vi "Termostato1.vi"() -> ()   [LabVIEW 2023]
uses:
  <vilib>/measure/NI_MABase.lvlib
panel:
  out "Coste del \nsuministro":dbl
  out "Potencia de \nla calefacción":dbl
  out "Consumo":bool
  out "Diferencia de temperatura":waveform(dbl)(graph)
  in  "offset":dbl format="%0.2p"
  in  "frequency":dbl=10.0 format="%0.2p"
  in  "amplitude":dbl=1.0 format="%0.2p"
  out "Temperatura\n Deseada":dbl format="%#.1f"
  out "Temperatura Actual":sgl(graph)
  out "Temp Ok":bool
  out "Suministro":bool
  in  "Slide":sgl(slide) scale=-5.0..60.0
  in  "stop":bool
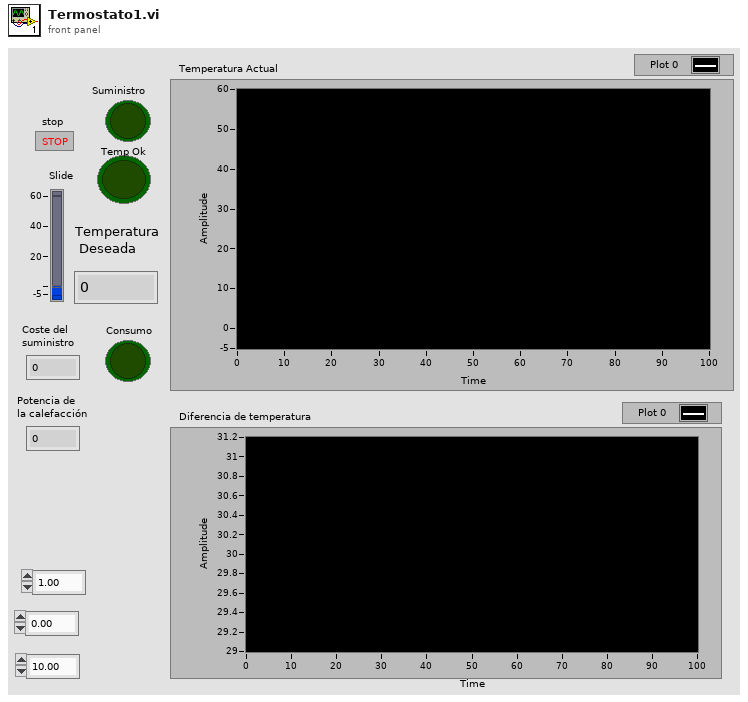
[diagram p1: front panel]
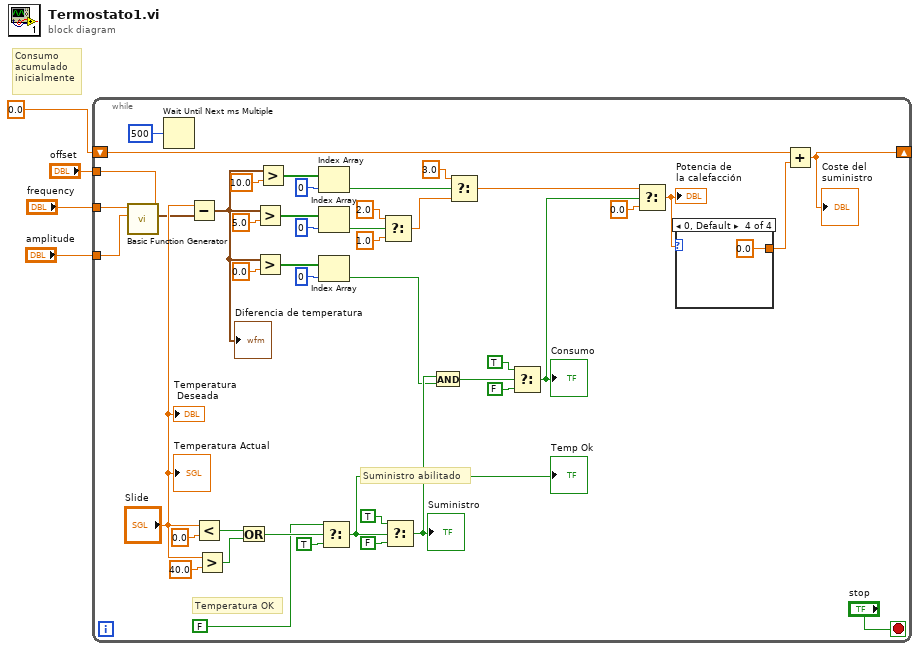
[diagram p0: block diagram]
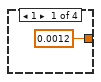
[diagram p2: hidden frame]
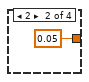
[diagram p3: hidden frame]
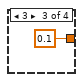
[diagram p4: hidden frame]
diagram:
  # "Consumo\nacumulado\ninicialmente"
  n1 = while {
    shift-right: [w6] -> _
    shift-left: 0.0 ("Numeric") -> [w7]
    tunnel: "offset" -> [w12]
    tunnel: "amplitude" -> [w11]
    tunnel: "frequency" -> [w10]
    stop <- "stop" stop-if-true
    # "Suministro abilitado"
    # "Temperatura OK"
    n2 = call <vilib>:"Basic Function Generator.vi"("offset"=w12, "amplitude"=w11, "frequency"=w10) -> ("signal out"=w9:waveform(dbl))  [unwired: 6 in, 2 out]
    n3 = Wait Until Next ms Multiple(millisecond multiple=u32 500 ("millisecond timer value")) -> ()  [unwired: 1 out]
    n4 = Subtract(x="Slide", y=w9) -> (x-y=w28:waveform(dbl))
    "Diferencia de temperatura" <- w28
    n5 = Less?(x="Slide", y=0.0) -> (x < y?=w39:bool)
    n6 = Greater?(x="Slide", y=40.0) -> (0:w47:bool)
    n7 = Or(x=w39, y=w47) -> (x .or. y?=w48:bool)
    n8 = Greater?(x=w28, y=5.0) -> (0:w26:bool[])
    n9 = Greater?(x=w28, y=0.0) -> (0:w31:bool[])
    n10 = Greater?(x=w28, y=10.0) -> (0:w23:bool[])
    n11 = Index Array(array=w23, index=0) -> (element=w22:bool)
    n12 = Index Array(array=w26, index=0) -> (element=w25:bool)
    n13 = Index Array(array=w31, index=0) -> (element=w32:bool)
    n14 = Select(t=FALSE, s=w48, f=TRUE) -> (s? t:f=w40:bool)
    "Temp Ok" <- w40
    n15 = Select(t=2.0, s=w25, f=1.0) -> (s? t:f=w18:dbl)
    n16 = Select(t=TRUE, s=w40, f=FALSE) -> (s? t:f=w35:bool)
    "Suministro" <- w35
    n17 = And(x=w35, y=w32) -> (x .and. y?=w34:bool)
    n18 = Select(t=3.0, s=w22, f=w18) -> (s? t:f=w16:dbl)
    n19 = Select(t=TRUE, s=w34, f=FALSE) -> (s? t:f=w14:bool)
    "Consumo" <- w14
    n20 = Select(t=w16, s=w14, f=0.0) -> (s? t:f=w8:dbl)
    "Potencia de \nla calefacción" <- w8
    n21 = case shown="0, Default" w8 {
      tunnel: [0.0012 ("f") 0.05 0.1 ("f") 0.0 ("f")] -> w5
      frame 1 {
      }
      frame 2 {
      }
      frame 3 {
      }
      frame 0, Default {
      }
    }
    n22 = Add(x=w7, y=w5) -> (x+y=w6:dbl)
    "Coste del \nsuministro" <- w6
    "Temperatura Actual" <- "Slide"
    "Temperatura\n Deseada" <- "Slide"
  }
